vi "Redo.vi"(8 "error in (no error)":errorcluster, 11 "Canvas in":refnum<class "Canvas.lvclass">) -> (0 "error out":errorcluster, 3 "Canvas out":refnum<class "Canvas.lvclass">)   [LabVIEW 2015, in "Canvas.lvclass"]
uses:
  Canvas.lvclass
  Canvas.lvclass/Canvas.ctl
  Graphic/Graphic.lvclass
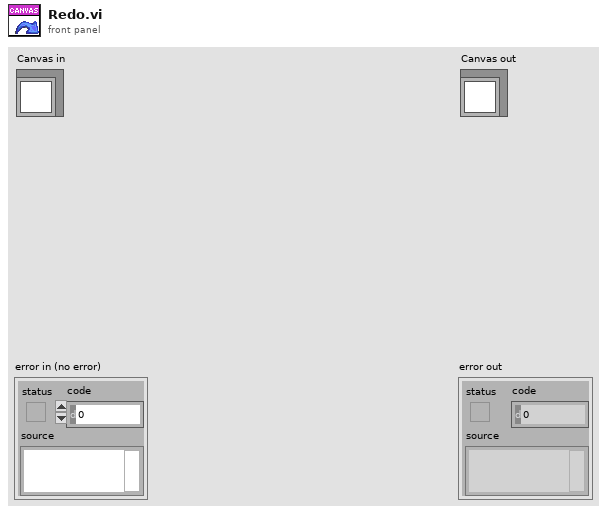
[diagram p1: front panel]
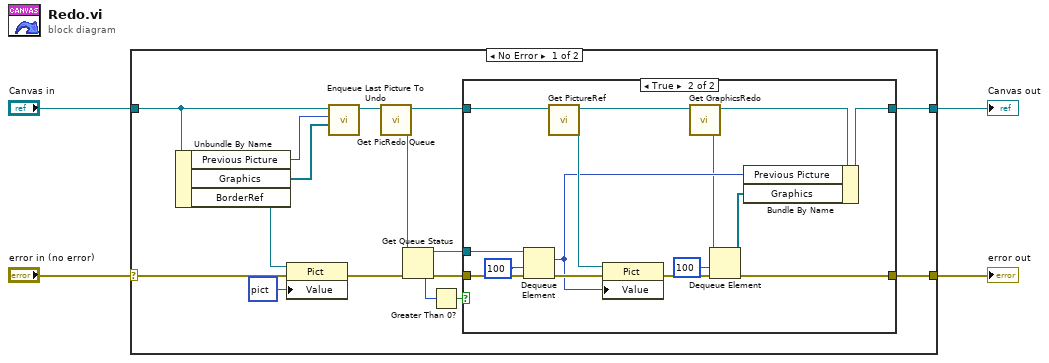
[diagram p0: block diagram]
diagram:
  n1 = case shown="No Error" "error in (no error)" {
    selector: "error in (no error)" -> [w18 w39]
    tunnel: [w11 w39] -> w3
    tunnel: [w19 w38] -> w1
    tunnel: "Canvas in" -> [w17 w38]
    frame No Error {
      n2 = Unbundle By Name(w17) -> ("Previous Picture"=w13:picture, "Graphics"=w12:refnum<class "Graphic.lvclass">[], "BorderRef"=w16:refnum<vi>)
      n3 = property class="Pict"(reference=w16, error in=w18, "Value"=picture data[5B]) -> (error out=w9:errorcluster)  [unwired: 1 out]
      n4 = call "Enqueue Last Picture To Undo.vi"("Graphics"=w12, "Last Picture"=w13, "Canvas in"=w17) -> ("Canvas out"=w14:refnum<class "Canvas.lvclass">)  [unwired: 7 in, 1 out]
      n5 = call "Get PicRedo Queue.vi"("Canvas in"=w14) -> ("PicRedo Queue"=w10:refnum<queue>, "Canvas out"=w20:refnum<class "Canvas.lvclass">)  [unwired: 8 in, 1 out]
      n6 = Get Queue Status(queue=w10, error in (no error)=w9) -> (queue out=w6:refnum<queue>, error out=w8:errorcluster, # elements in queue=w7:i32)  [unwired: 1 in, 5 out]
      n7 = Greater Than 0?(x=w7) -> (x > 0?=w5:bool)
      n8 = case shown="True" w5 {
        tunnel: w20 -> [w22 w37]
        tunnel: [w22 w32] -> w19
        tunnel: [w21 w27] -> w11
        tunnel: w8 -> [w21 w24]
        tunnel: w6 -> [_ w23]
        frame False {
        }
        frame True {
          n9 = Dequeue Element(queue=w23, timeout in ms (-1)=100, error in (no error)=w24) -> (element=w31:picture, error out=w33:errorcluster)  [unwired: 2 out]
          n10 = call "Get PictureRef.vi"("Canvas in"=w37) -> ("PictureRef"=w34:refnum<vi>, "Canvas out"=w35:refnum<class "Canvas.lvclass">)  [unwired: 8 in, 1 out]
          n11 = property class="Pict"(reference=w34, error in=w33, "Value"=w31) -> (error out=w28:errorcluster)  [unwired: 1 out]
          n12 = call "Get GraphicsRedo.vi"("Canvas in"=w35) -> ("GraphicsRedo"=w26:refnum<queue>, "Canvas out"=w30:refnum<class "Canvas.lvclass">)  [unwired: 8 in, 1 out]
          n13 = Dequeue Element(queue=w26, timeout in ms (-1)=100, error in (no error)=w28) -> (element=w25:refnum<class "Graphic.lvclass">[], error out=w27:errorcluster)  [unwired: 2 out]
          n14 = Bundle By Name(cluster=w30, "Previous Picture"=w31, "Graphics"=w25) -> (w32:refnum<class "Canvas.lvclass">)
        }
      }
    }
    frame Error {
    }
  }
  "error out" <- w3
  "Canvas out" <- w1
